vi "Broadcast Unfiltered Debug Data.vi"(8 "error in (no error)":errorcluster, 11 "Debugger in":refnum<class "Debugger.lvclass">) -> (0 "error out":errorcluster, 3 "Debugger out":refnum<class "Debugger.lvclass">)   [LabVIEW 2020, in "Debugger.lvclass"]
uses:
  Debugger.lvclass
  Debugger.lvclass/Debugger.ctl
  Process/Debug Process.lvclass
  C:/Users/anton/Documents/GitHub/triarc-debugger/source/Process/Debug Process.lvclass
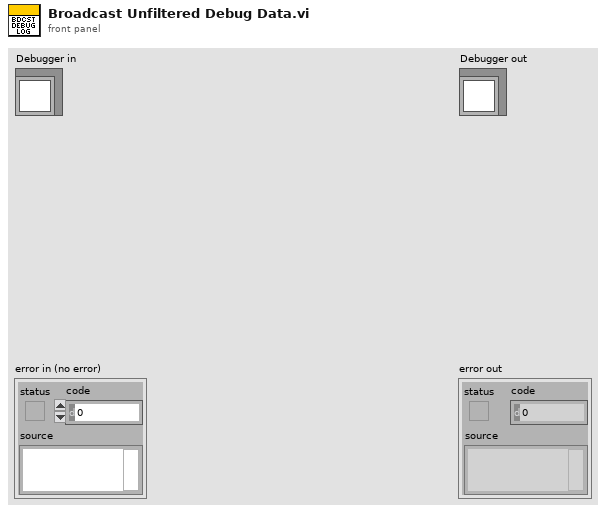
[diagram p1: front panel]
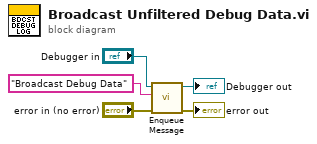
[diagram p0: block diagram]
diagram:
  n1 = call "Enqueue Message.vi"("error in (no error)"="error in (no error)", "Message"="Broadcast Debug Data", "Process In"="Debugger in") -> ("error out"=→"error out":errorcluster, "Process Out"=→"Debugger out":refnum<class "Debugger.lvclass">)  [unwired: 7 in]
